vi "Get PE Specification.vi"(8 "error in (no error)":errorcluster, 11 "RandomNumberLogger Controller in":refnum<class "RandomNumberLogger Controller.lvclass">) -> (0 "error out":errorcluster, 2 "PE Specification":T1, 3 "RandomNumberLogger Controller out":refnum<class "RandomNumberLogger Controller.lvclass">)   [LabVIEW 2020, in "RandomNumberLogger.lvlib" / "RandomNumberLogger Controller.lvclass"]
doc: "<b>Get PE Specification</b>\nThis method combines the three pieces of the PE Specication:\n - Output Streams: The outputs from this plugin\n - Type ID: The unique ID for this plugin\n - Parameters: All of the parameters that can be configured for this plugin\n\nThis informatoin is passed out to the <b>Configuration Utility</b> via the plugin XML file."
uses:
  RandomNumberLogger Controller.lvclass
  <vilib>/FlexLogger/SDK/PluginSDK.lvlibp/PEFClasses/SDK/Processing Element Specification/PE Specification.ctl
  <vilib>/FlexLogger/SDK/PluginSDK.lvlibp/PEFClasses/SDK/Processing Element Specification/Parameter Specification.ctl
  <vilib>/FlexLogger/SDK/PluginSDK.lvlibp/PEFClasses/SDK/Processing Element Specification/Parameter Type.ctl
  <vilib>/FlexLogger/SDK/PluginSDK.lvlibp/PEFClasses/SDK/Processing Element Specification/Stream Specification.ctl
  RandomNumberLogger Controller.lvclass/RandomNumberLogger Controller.ctl
  Read Output Streams.vi
  PE/Get Configuration Version.vi
  <vilib>/ADAS Record/Utilities/Config/Data Converter/Data Container and Version to JSON.vi
  PE/RandomNumberLogger.lvclass
  <vilib>/FlexLogger/SDK/PluginSDK.lvlibp/PEFClasses/SDK/Processing Element Specification/Processing Element Specification.lvclass
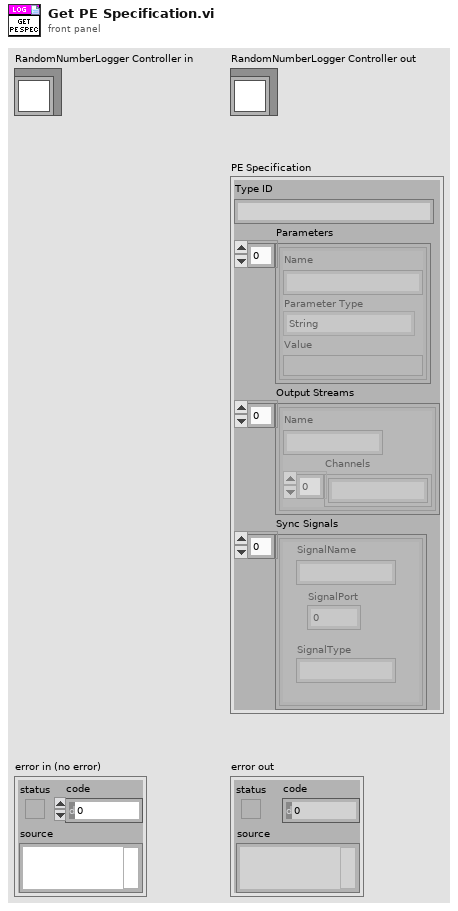
[diagram p1: front panel]
types:
  T1 = typedef "PluginSDK.lvlibp/Processing Element Specification.lvclass/PE Specification.ctl" = cluster{"Type ID":string, "Parameters":T2[], "Output Streams":T4[], "Sync Signals":cluster{"SignalName":string, "SignalPort":i32, "SignalType":string}[]}
  T2 = typedef "PluginSDK.lvlibp/Processing Element Specification.lvclass/Parameter Specification.ctl" = cluster{"Name":string, "Parameter Type":T3, "Value":variant}
  T3 = typedef "PluginSDK.lvlibp/Processing Element Specification.lvclass/Parameter Type.ctl" = enum16{"String", "JSON", "Double", "Int32", "Boolean"}
  T4 = typedef "PluginSDK.lvlibp/Processing Element Specification.lvclass/Stream Specification.ctl" = cluster{"Name":string, "Channels":string[]}
  T5 = typedef "RandomNumberLogger.lvlib/RandomNumberLogger.lvclass/Configuration.ctl" = cluster{"Parameter1":string}
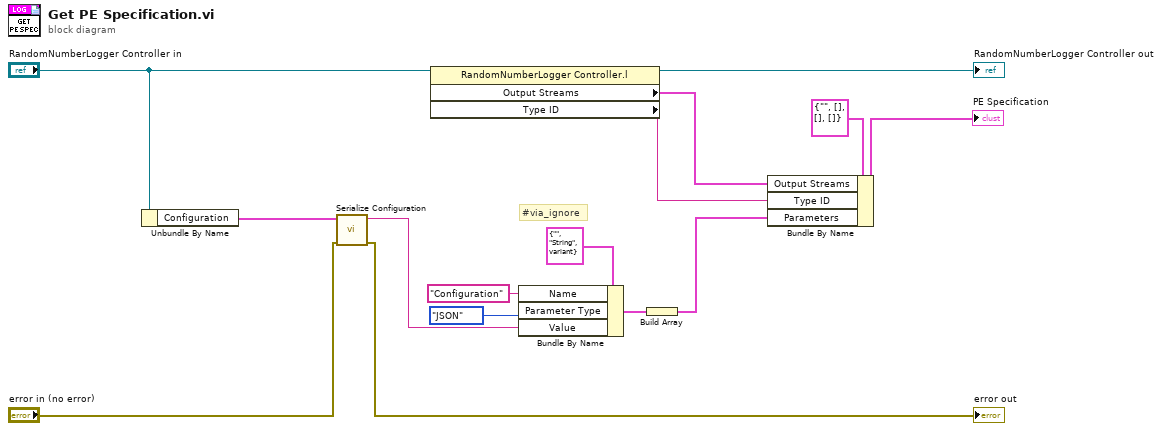
[diagram p0: block diagram]
diagram:
  # "#via_ignore"
  n1 = Unbundle By Name("RandomNumberLogger Controller in") -> ("Configuration"=w13:T5)
  n2 = call "Serialize Configuration.vi"("error in (no error)"="error in (no error)", "Configuration"=w13) -> ("error out"=→"error out":errorcluster, "Serialized Configuration"=w9:string)  [unwired: 8 in]
  n3 = property on="Property Node" class="RandomNumberLogger Controller.l"(reference="RandomNumberLogger Controller in") -> (reference out=→"RandomNumberLogger Controller out":refnum<class "RandomNumberLogger Controller.lvclass">, "Output Streams"=w5:T4[], "Type ID"=w4:string)  [unwired: 1 in, 1 out]
  n4 = Bundle By Name(cluster=T2 {"Name"="", "Parameter Type"=enum."String", "Value"=variant} ("Parameter"), "Name"="Configuration", "Parameter Type"=Parameter_Type."JSON", "Value"=w9) -> (w8:T2)
  n5 = Build Array(w8) -> (w7:T2[])
  n6 = Bundle By Name(cluster=T1 {"Type ID"="", "Parameters"=[], "Output Streams"=[], "Sync Signals"=[]} ("PE Specification"), "Output Streams"=w5, "Type ID"=w4, "Parameters"=w7) -> (→"PE Specification":T1)
